vi "Initailize.vi"(8 "error in (no error)":errorcluster, 9 "zeromq.lvlib:ZeroMQ Context":refnum<class "zmq_context.lvclass">, 10 "Name":string, 11 "Channel Rep in":refnum<class "Channel Rep.lvclass">) -> (0 "error out":errorcluster, 3 "Channel Rep out":refnum<class "Channel Rep.lvclass">)   [LabVIEW 2018, in "Channel Rep.lvclass"]
uses:
  Channel Rep.lvclass
  <vilib>/addons/zeromq/zmq_context.lvclass
  Communication Channel/Communication Channel Folder/Communication Channel.lvclass
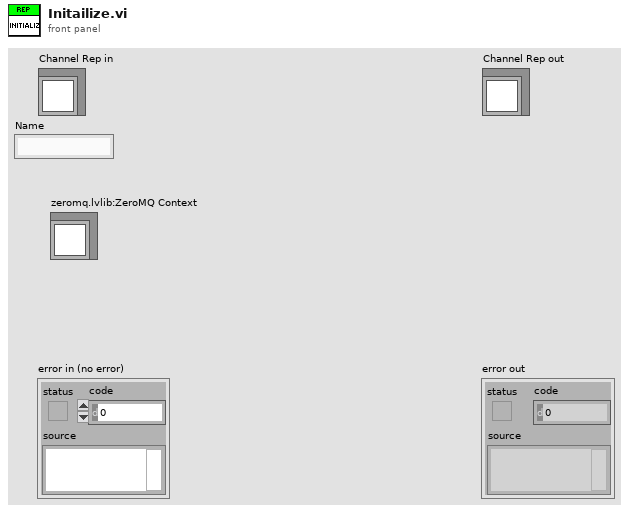
[diagram p1: front panel]
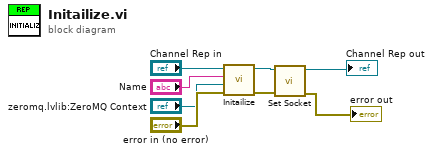
[diagram p0: block diagram]
diagram:
  n1 = call-parent "Initailize.vi"("error in (no error)"="error in (no error)", "zeromq.lvlib:ZeroMQ Context"="zeromq.lvlib:ZeroMQ Context", "Name"="Name", "Communication Channel in"="Channel Rep in") -> ("error out"=w3:errorcluster, "Communication Channel out"=w4:refnum<class "Channel Rep.lvclass">)  [unwired: 6 in]
  n2 = call-dynamic "Set Socket.vi"("error in (no error)"=w3, "Channel Rep in"=w4) -> ("error out"=→"error out":errorcluster, "Channel Rep out"=→"Channel Rep out":refnum<class "Channel Rep.lvclass">)  [unwired: 8 in]
